vi "_AcquireSingleScan.vi"() -> ()   [LabVIEW 2024]
uses:
  X-Scales.ctl
  ff6a1ae8-2aae-4c4f-bccd-18872fa50bd4.vi
panel:
  in  "Plot Data":bool
  in  "New Scan":bool
  out "Finding DUT Length":bool
  in  "Find DUT Length?":bool
  in  "filter data?":bool
  out "Graph":T1(graph) caption="Insertion Loss"
  in  "X-axis units":T2
  in  "Group Index":dbl=1.5 format="%.2f"
  in  "res BW (GHz)":dbl format="%.2f"
  out "genOutput":dbl[](array[numeric]) format="%.2f"
  in  "Graph Sel":u16(ring) items=["Insertion Loss", "Group Delay", "Chromatic Dispersion", "Polarization Dependent Loss", "Polarization Mode Dispersion", "Linear Phase Deviation", "Quadratic Phase Deviation", "Jones Matrix Element Amplitudes", "Jones Matrix Element Phases", "Time Domain Amplitude", "Time Domain Wavelength", "Min/Max Loss", "Second Order PMD", "Phase Ripple Linear", "Phase Ripple Quadratic"]
  out "error":errorcluster
  in  "Length of DUT (m)":dbl=3.0 format="%.3f"
  in  "Center WL":dbl=1550.0 caption="Center Wavelength (nm)" step=0.01 format="%.2f"
  in  "Meas Type":u16(ring)=1 caption="Type of Measurement" items=["Reflection", "Transmission"]
  in  "WL Range":u16(ring)=2 caption="Wavelength Range (nm)" items=["0.63", "1.27", "2.54", "5.09", "10.22", "20.58", "41.72", "85.78"]
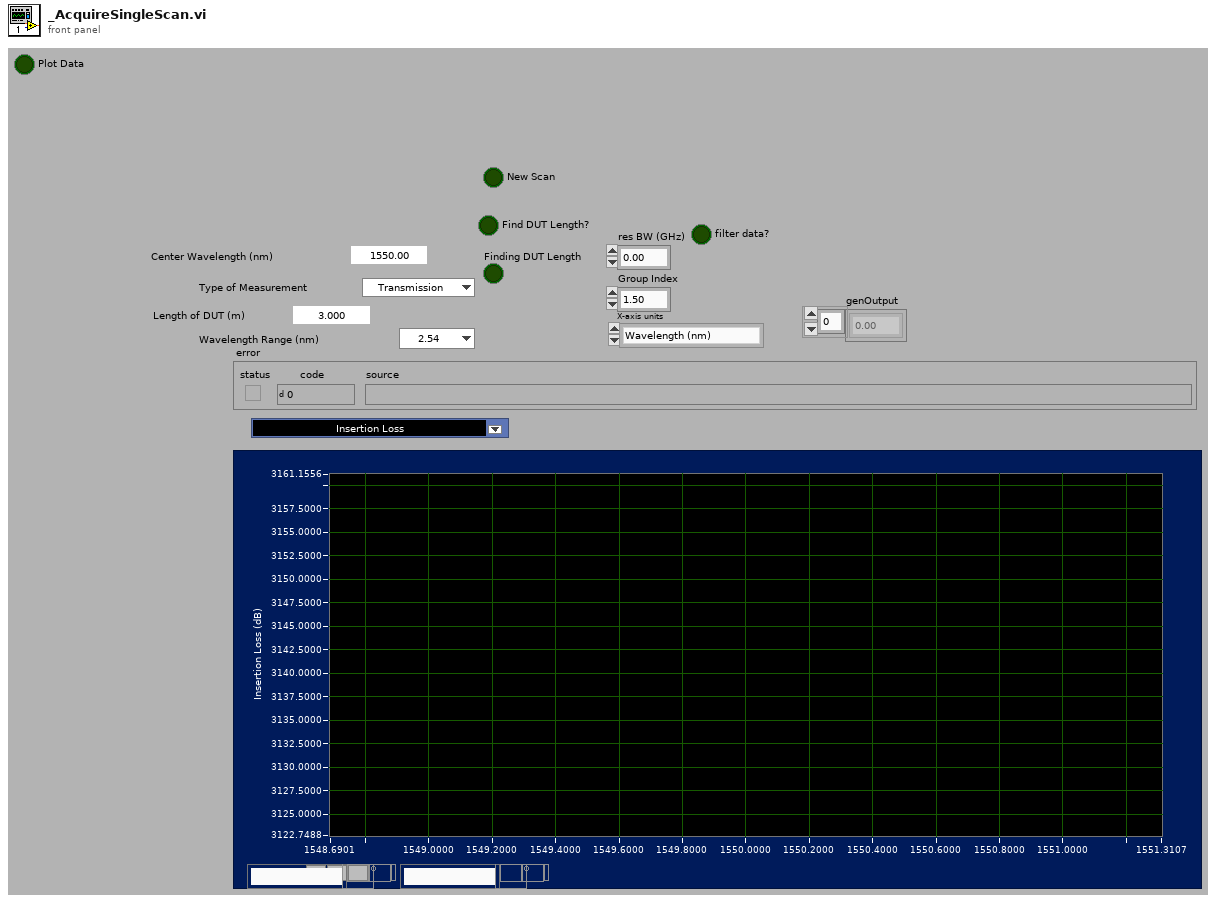
[diagram p1: front panel]
types:
  T1 = cluster{"Array Constant":dbl[], "Array Constant":dbl[]}[]
  T2 = typedef "X-Scales.ctl" = enum16{"Wavelength (nm)", "Gigahertz (GHz)", "Terahertz (THz)", "Time (ns)", "Length (m)"}
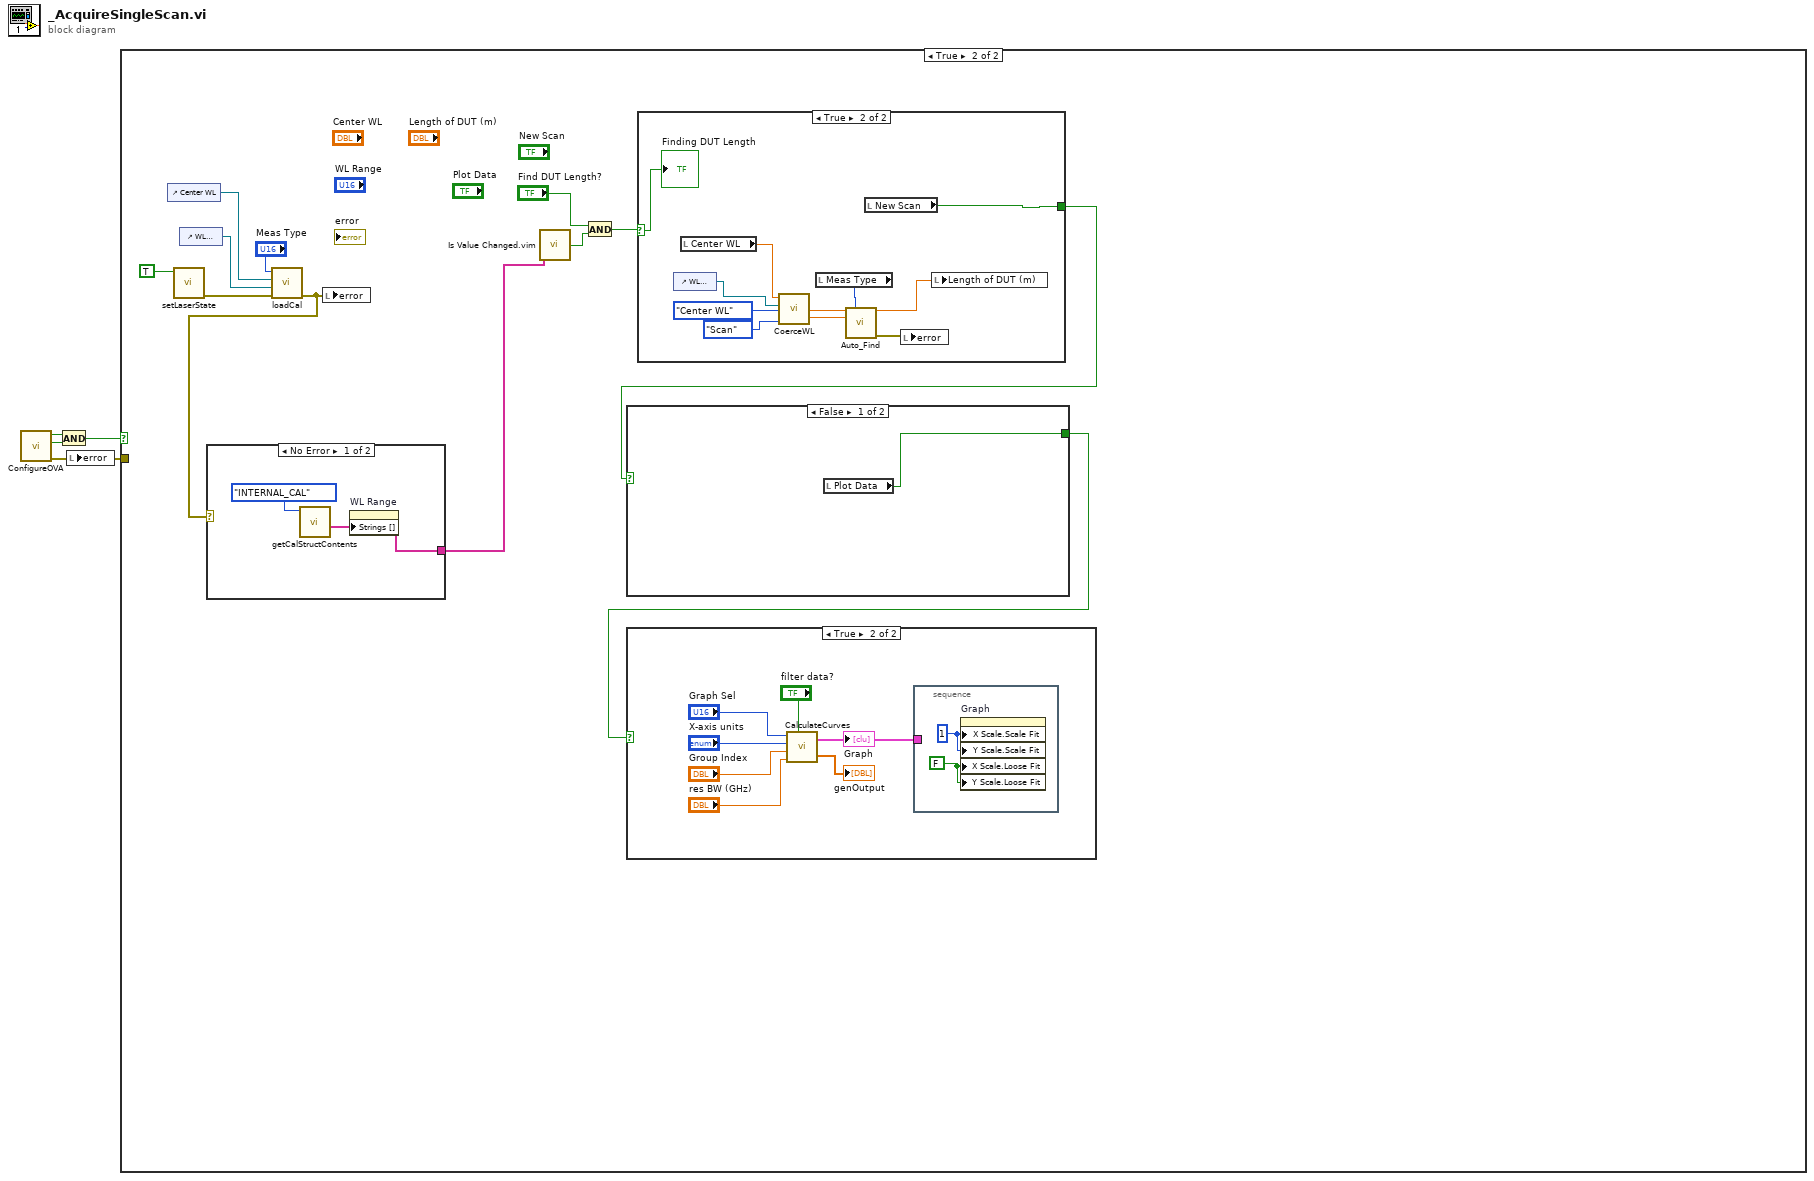
[diagram p0: block diagram]
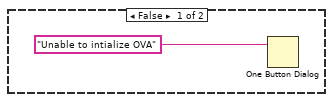
[diagram p2: hidden frame]
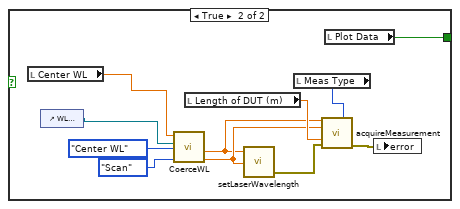
[diagram p4: hidden frame]
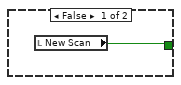
[diagram p5: hidden frame]
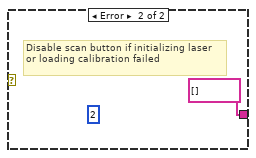
[diagram p6: hidden frame]
diagram:
  n1 = call "ConfigureOVA.vi"() -> ("error out"=w1:errorcluster, "Cfg OK?"=w3:bool, "instrFound"=w4:bool)  [unwired: 4 in, 1 out]
  n2 = And(x=w4, y=w3) -> (x .and. y?=w2:bool)
  n3 = local write "error"(w1) -> ()
  n4 = case shown="True" w2 {
    tunnel: w1 -> [_ _]
    frame False {
      n5 = One Button Dialog(message="Unable to intialize OVA") -> ()  [unwired: 1 in, 1 out]
    }
    frame True {
      n6 = control-ref of="Center WL"() -> (w12:refnum<vi>)
      n7 = call "setLaserState.vi"("New Laser Status"=TRUE) -> ("error out"=w16:errorcluster)  [unwired: 6 in]
      n8 = control-ref of="WL Range"() -> (w14:refnum<vi>)
      n9 = call "loadCal.vi"("error in (no error)"=w16, "Wavelength Range (nm)"=w14, "Center WL (nm)"=w12, "Type of Measurement"="Meas Type") -> ("error out"=w13:errorcluster)  [unwired: 6 in, 1 out]
      n10 = case shown="No Error" w13 {
        tunnel: [w52 string[] [] ("Range Strings")] -> w9
        frame No Error {
          n11 = call "getCalStructContents.vi"("calType"=enum16{"INTERNAL_CAL", "FULL_CAL"}."INTERNAL_CAL" ("Enum")) -> ("Range Strings"=w52:string[])  [unwired: 7 in, 3 out]
          n12 = property on="WL Range" class="Ring (strict)"("Strings []"=w52) -> ()  [unwired: 2 in, 2 out]
        }
        frame Error {
          (unwired) u8 2 ("Disabled")
          # "Disable scan button if initializing laser or loading calibration failed"
        }
      }
      n13 = local write "error"(w13) -> ()
      n14 = call "Is Value Changed.vim"("value"=w9) -> ("changed or first call?"=w8:bool)
      n15 = And(x="Find DUT Length?", y=w8) -> (x .and. y?=w10:bool)
      n16 = case shown="True" w10 {
        selector: w10 -> [_ w50]
        tunnel: [w39 w40] -> w7
        frame False {
          n17 = local read "New Scan"() -> (w39:bool)
        }
        frame True {
          n18 = control-ref of="WL Range"() -> (w48:refnum<vi>)
          n19 = local read "Center WL"() -> (w49:dbl)
          n20 = call "CoerceWL.vi"("Parameter Type"=enum16{"Calibration", "Scan"}."Scan", "wlType"=enum16{"Center WL", "Start WL"}."Center WL", "Wavelength Range (nm)"=w48, "Start/Center Wavelength (nm)"=w49) -> ("end WL (nm)"=w46:dbl, "start WL (nm)"=w45:dbl)  [unwired: 4 in, 2 out]
          n21 = local read "Meas Type"() -> (w44:u16)
          n22 = call "Auto_Find.vi"("Start WL -- nm"=w45, "Type of Measurement"=w44, "End WL -- nm"=w46) -> ("Length of DUT (m)"=w41:dbl, "error out"=w47:errorcluster)  [unwired: 10 in, 1 out]
          n23 = local read "New Scan"() -> (w40:bool)
          n24 = local write "error"(w47) -> ()
          n25 = local write "Length of DUT (m)"(w41) -> ()
          "Finding DUT Length" <- w50
        }
      }
      n26 = case shown="False" w7 {
        tunnel: [w27 w28] -> w6
        frame False {
          n27 = local read "Plot Data"() -> (w27:bool)
        }
        frame True {
          n28 = local read "Center WL"() -> (w36:dbl)
          n29 = control-ref of="WL Range"() -> (w35:refnum<vi>)
          n30 = call "CoerceWL.vi"("Parameter Type"=enum16{"Calibration", "Scan"}."Scan", "wlType"=enum16{"Center WL", "Start WL"}."Center WL", "Wavelength Range (nm)"=w35, "Start/Center Wavelength (nm)"=w36) -> ("end WL (nm)"=w32:dbl, "start WL (nm)"=w31:dbl)  [unwired: 4 in, 2 out]
          n31 = local read "Length of DUT (m)"() -> (w37:dbl)
          n32 = call "setLaserWavelength.vi"("End Wavelength (nm)"=w32, "Start Wavelength (nm)"=w31) -> ("error out"=w33:errorcluster)  [unwired: 2 in, 1 out]
          n33 = local read "Meas Type"() -> (w34:u16)
          n34 = call "acquireMeasurement.vi"("startWL (nm)"=w31, "Type of Measurement"=w34, "endWL (nm)"=w32, "dutLength (m)"=w37, "error in (no error)"=w33) -> ("error out"=w38:errorcluster)  [unwired: 5 in, 5 out]
          n35 = local read "Plot Data"() -> (w28:bool)
          n36 = local write "error"(w38) -> ()
        }
      }
      n37 = case shown="True" w6 {
        frame False {
        }
        frame True {
          n38 = call "CalculateCurves.vi"("Graph Sel"="Graph Sel", "X-axis units"="X-axis units", "Group Index"="Group Index", "res BW (GHz)"="res BW (GHz)", "filter?"="filter data?") -> ("Graph Data"=w23:cluster{dbl[], dbl[]}[], "genOutput"=→"genOutput":dbl[])
          "Graph" <- w23
          n39 = stacked-sequence {
            tunnel: w23 -> [_]
            frame #0 {
              w25 = FALSE ("X Scale.Loose Fit")
              w26 = u8 1 ("X Scale.Scale Fit")
              n40 = property on="Graph" class="XYGraph (strict)"("X Scale.Scale Fit"=w26, "Y Scale.Scale Fit"=w26, "X Scale.Loose Fit"=w25, "Y Scale.Loose Fit"=w25) -> ()  [unwired: 2 in, 2 out]
            }
          }
        }
      }
    }
  }
